vi "Get_Time_Stamp.vi"(11 "error in":errorcluster) -> (3 "error out":errorcluster, 4 "current time":timestamp)   [LabVIEW 2018]
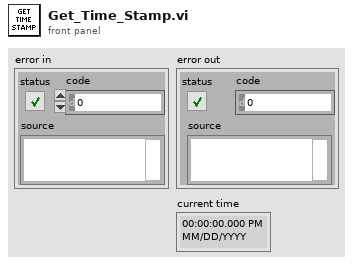
[diagram p1: front panel]
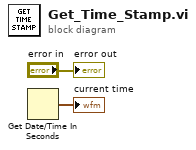
[diagram p0: block diagram]
diagram:
  n1 = Get Date/Time In Seconds() -> (seconds since 1Jan1904=→"current time":timestamp)
  "error out" <- "error in"
